vi "Build Tree Data.vi"(8 "error in (no error)":errorcluster, 11 "Test Executive Builder Model in":refnum<class "Test Executive Builder Model.lvclass">) -> (0 "error out":errorcluster, 1 "Tree Data":T1(array[cluster]), 3 "Test Executive Builder Model out":refnum<class "Test Executive Builder Model.lvclass">)   [LabVIEW 2017, in "Test Executive Builder Model.lvclass"]
uses:
  Test Executive Builder Model.lvclass
  <vilib>/gpm_packages/@cs/test-executive/Source/Test Executive/TestExecutive Ref/TestExecutive Ref.lvclass
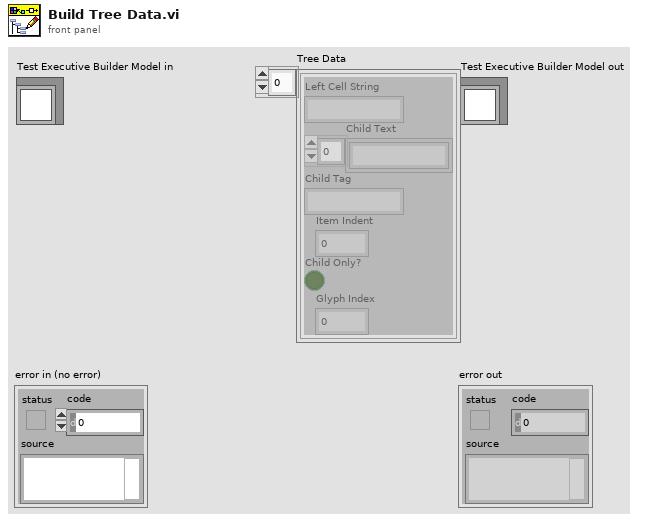
[diagram p1: front panel]
types:
  T1 = cluster{"Left Cell String":string, "Child Text":string[], "Child Tag":string, "Item Indent":i32, "Child Only?":bool, "Glyph Index":i32}[]
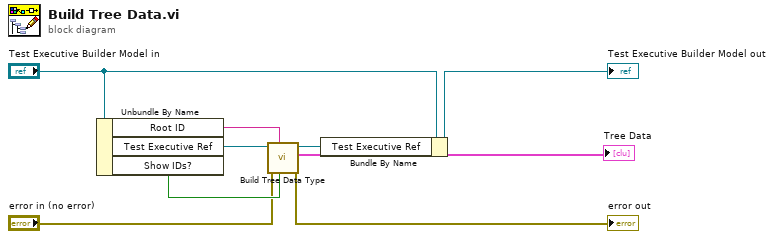
[diagram p0: block diagram]
diagram:
  n1 = Unbundle By Name("Test Executive Builder Model in") -> ("Root ID"=w8:string, "Test Executive Ref"=w9:refnum<data-value>, "Show IDs?"=w7:bool)
  n2 = call <vilib>:"Build Tree Data Type.vi"("Show IDs (True)"=w7, "Test ID"=w8, "error in (no error)"="error in (no error)", "Test Executive Ref"=w9) -> ("error out"=→"error out":errorcluster, "Tree Data"=→"Tree Data":T1, "Test Executive Ref out"=w1:refnum<data-value>)  [unwired: 5 in]
  n3 = Bundle By Name(cluster="Test Executive Builder Model in", "Test Executive Ref"=w1) -> (→"Test Executive Builder Model out":refnum<class "Test Executive Builder Model.lvclass">)
